vi "ClusterToDescriptiveStringGeneral.vi"(8 "error in":errorcluster, 11 "Cluster In":refnum<vi>) -> (0 "error out":errorcluster, 3 "String":string)   [LabVIEW 2023]
doc: "This VI turns a cluster (from reference) into a human/machine readable string."
panel:
  out "data":dbl[](array[numeric])
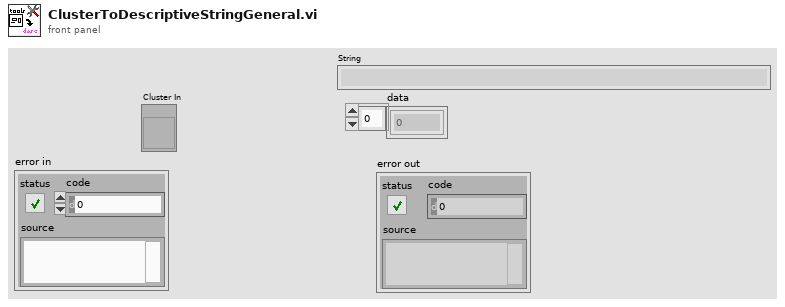
[diagram p1: front panel]
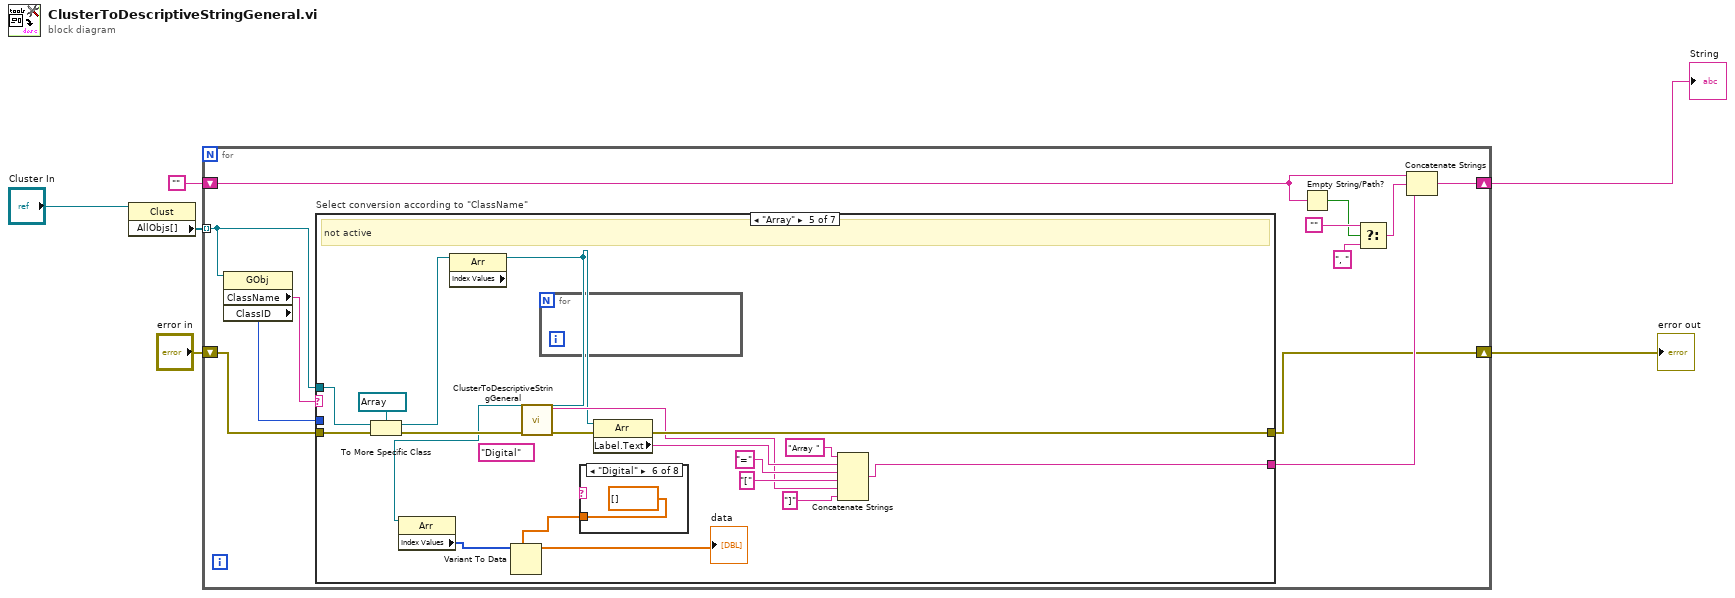
[diagram p0: block diagram]
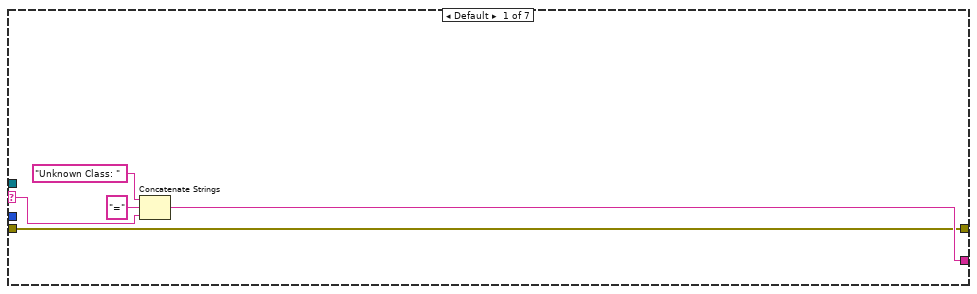
[diagram p2: hidden frame]
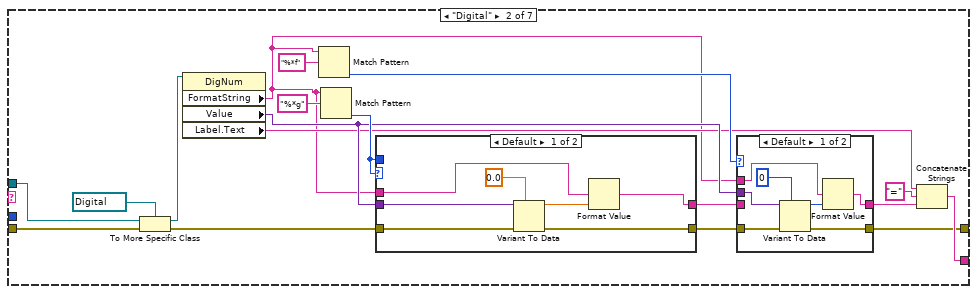
[diagram p3: hidden frame]
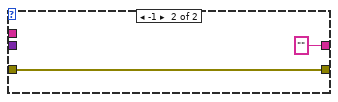
[diagram p5: hidden frame]
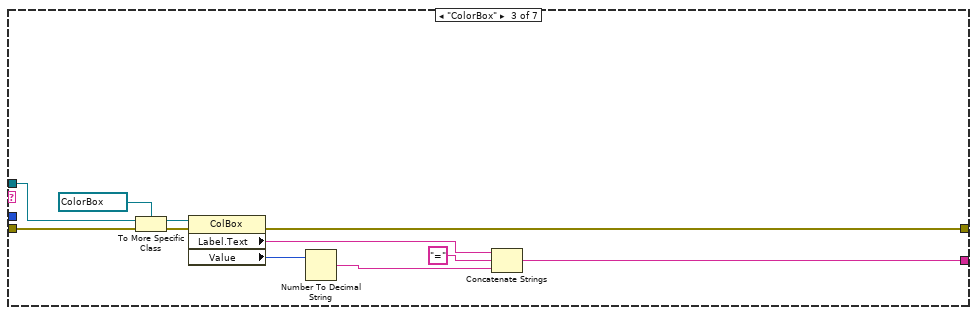
[diagram p6: hidden frame]
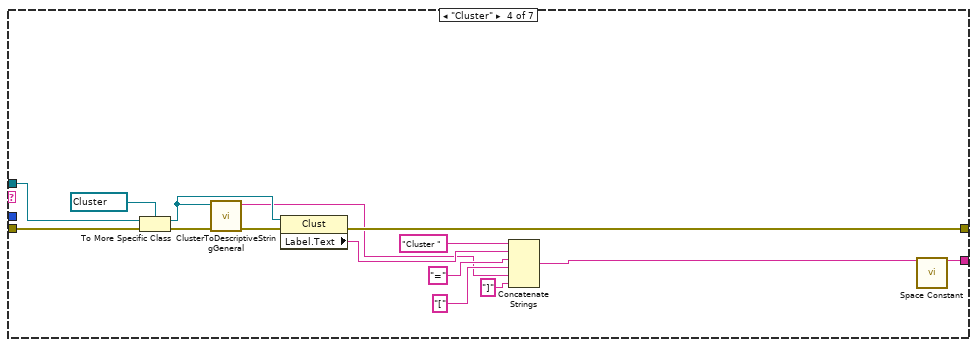
[diagram p7: hidden frame]
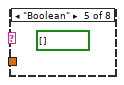
[diagram p12: hidden frame]
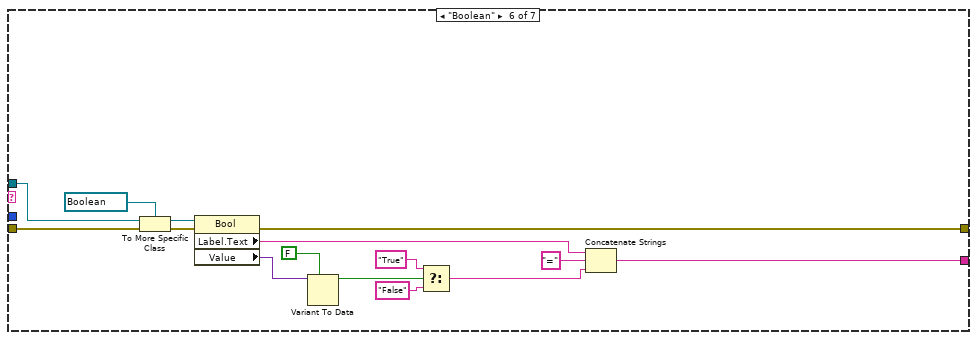
[diagram p15: hidden frame]
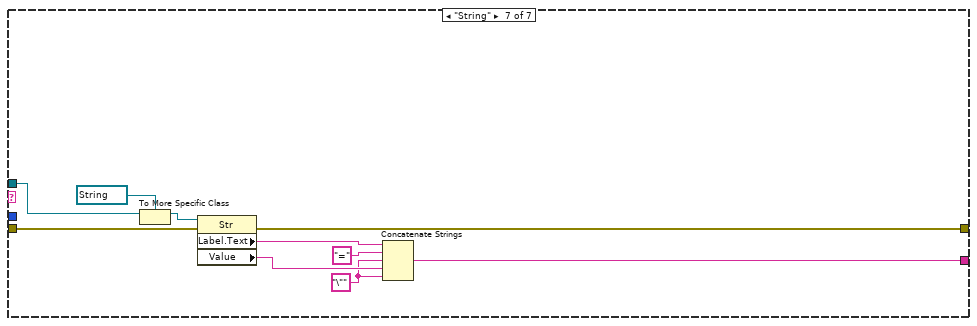
[diagram p16: hidden frame]
diagram:
  n1 = property on="Property Node" class="Clust"(reference="Cluster In") -> ("AllObjs[]"=w2:refnum<vi>[])  [unwired: 1 in, 2 out]
  n2 = for {
    tunnel: w2 -> [w17] mode=indexing
    shift-right: [w18] -> w6
    shift-left: "" ("Empty String Constant") -> [w8]
    shift-right: [w11] -> w3
    shift-left: "error in" -> [w10]
    n3 = property on="Property Node" class="GObj"(reference=w17) -> ("ClassName"=w15:string, "ClassID"=w16:u32)  [unwired: 1 in, 2 out]
    n4 = case "Select conversion according to \"ClassName\"" shown="\"Array\"" w15 {
      selector: w15 -> [w21 _ _ _ _ _ _]
      tunnel: [w20 w31 w66 w82 w100 w115 w126] -> w14
      tunnel: w17 -> [_ w41 w70 w84 w102 w118 w128]
      tunnel: w16 -> [_ _ _ _ _ _ _]
      tunnel: [w19 w25 w62 w79 w98 w106 w120] -> w11
      tunnel: w10 -> [w19 w28 w60 w78 w97 w104 w119]
      frame Default {
        n5 = Concatenate Strings("Unknown Class: ", "=", w21) -> (w20:string)
      }
      frame "Digital" {
        n6 = To More Specific Class(target class=refnum<vi> refnum ("567"), reference=w41, error in=w28) -> (specific class reference=w40:refnum<vi>, error out=w27:errorcluster)
        n7 = property on="Property Node" class="DigNum"(reference=w40) -> ("FormatString"=w30:string, "Value"=w37:variant, "Label.Text"=w33:string)  [unwired: 1 in, 2 out]
        n8 = Match Pattern(string=w30, regular expression="%*f") -> (offset past match=w34:i32)  [unwired: 1 in, 3 out]
        n9 = Match Pattern(string=w30, regular expression="%*g") -> (offset past match=w39:i32)  [unwired: 1 in, 3 out]
        n10 = case shown="Default" w39 {
          tunnel: w39 -> [_ _]
          tunnel: w37 -> [w57 _]
          tunnel: [w55 "" ("output string")] -> w38
          tunnel: w30 -> [w54 _]
          tunnel: w27 -> [w53 w58]
          tunnel: [w52 w58] -> w26
          frame Default {
            n11 = Variant To Data(error in=w53, type=0.0, Variant=w57) -> (data=w56:dbl, error out=w52:errorcluster)
            n12 = Format Value(format string=w54, value (0)=w56) -> (output string=w55:string)  [unwired: 1 in]
          }
          frame -1 {
          }
        }
        n13 = case shown="Default" w34 {
          tunnel: w37 -> [w48 _]
          tunnel: w38 -> [_ w50]
          tunnel: [w46 w50] -> w32
          tunnel: w30 -> [w45 _]
          tunnel: w26 -> [w44 w49]
          tunnel: [w43 w49] -> w25
          frame Default {
            n14 = Variant To Data(error in=w44, type=0, Variant=w48) -> (data=w47:i32, error out=w43:errorcluster)
            n15 = Format Value(format string=w45, value (0)=w47) -> (output string=w46:string)  [unwired: 1 in]
          }
          frame -1 {
          }
        }
        n16 = Concatenate Strings(w33, "=" ("string"), w32) -> (w31:string)
      }
      frame "ColorBox" {
        n17 = To More Specific Class(target class=refnum<vi> refnum ("Left"), reference=w70, error in=w60) -> (specific class reference=w69:refnum<vi>, error out=w61:errorcluster)
        n18 = property on="Property Node" class="ColBox"(reference=w69, error in=w61) -> (error out=w62:errorcluster, "Label.Text"=w67:string, "Value"=w64:u32)  [unwired: 1 out]
        n19 = Number To Decimal String(number=w64) -> (decimal integer string=w68:string)  [unwired: 1 in]
        n20 = Concatenate Strings(w67, "=" ("string"), w68) -> (w66:string)
      }
      frame "Cluster" {
        n21 = To More Specific Class(target class=refnum<vi> refnum ("Left"), reference=w84, error in=w78) -> (specific class reference=w76:refnum<vi>, error out=w77:errorcluster)
        n22 = call "ClusterToDescriptiveStringGeneral.vi"("error in"=w77, "Cluster In"=w76) -> ("error out"=w75:errorcluster, "String"=w73:string)  [unwired: 8 in]
        n23 = property on="Property Node" class="Clust"(reference=w76, error in=w75) -> (error out=w79:errorcluster, "Label.Text"=w83:string)  [unwired: 1 out]
        n24 = Concatenate Strings("Cluster " ("string"), w83, "=" ("string"), "[" ("string"), w73, "]" ("string")) -> (w82:string)
        n25 = call <vilib>:"Space Constant.vi"() -> ()  [unwired: 1 out]
      }
      frame "Array" {
        (unwired) "Digital" ("Combo Box")
        # "not active"
        n26 = To More Specific Class(target class=refnum<vi> refnum ("Left"), reference=w102, error in=w97) -> (specific class reference=w89:refnum<vi>, error out=w96:errorcluster)
        n27 = property on="Property Node" class="Arr" props=["Index Values"](reference=w89) -> (reference out=w88:refnum<vi>)  [unwired: 1 in, 2 out]
        n28 = property on="Property Node" class="Arr"(reference=w88) -> ("Index Values"=w87:u32[])  [unwired: 1 in, 2 out]
        n29 = call "ClusterToDescriptiveStringGeneral.vi"("error in"=w96) -> ("error out"=w95:errorcluster, "String"=w93:string)  [unwired: 9 in]
        n30 = for {
        }
        n31 = case shown="\"Digital\"" {
          selector: _ -> [_ _ _ _ _ _ _ _]
          tunnel: [_ _ _ _ _ dbl[] [] _ _] -> w86
          frame "False", Default {
          }
          frame "True" {
          }
          frame "String" {
          }
          frame "ColorBox" {
          }
          frame "Boolean" {
            (unwired) bool[] []
          }
          frame "Digital" {
          }
          frame "Array" {
          }
          frame "Cluster" {
          }
        }
        n32 = Variant To Data(type=w86, Variant=w87) -> (data=→"data":dbl[])  [unwired: 1 in, 1 out]
        n33 = property on="Property Node" class="Arr"(reference=w88, error in=w95) -> (error out=w98:errorcluster, "Label.Text"=w101:string)  [unwired: 1 out]
        n34 = Concatenate Strings("Array " ("string"), w101, "=" ("string"), "[" ("string"), w93, "]" ("string")) -> (w100:string)
      }
      frame "Boolean" {
        n35 = To More Specific Class(target class=refnum<vi> refnum ("Left"), reference=w118, error in=w104) -> (specific class reference=w117:refnum<vi>, error out=w105:errorcluster)
        n36 = property on="Property Node" class="Bool"(reference=w117, error in=w105) -> (error out=w106:errorcluster, "Label.Text"=w116:string, "Value"=w112:variant)  [unwired: 1 out]
        n37 = Variant To Data(type=FALSE ("x = y?"), Variant=w112) -> (data=w110:bool)  [unwired: 1 in, 1 out]
        n38 = Select(t="True" ("Label.Text"), s=w110, f="False" ("Label.Text")) -> (s? t:f=w107:string)
        n39 = Concatenate Strings(w116, "=" ("string"), w107) -> (w115:string)
      }
      frame "String" {
        w123 = "\"" ("string")
        n40 = To More Specific Class(target class=refnum<vi> refnum ("Numeric"), reference=w128) -> (specific class reference=w127:refnum<vi>)  [unwired: 1 in, 1 out]
        n41 = property on="Property Node" class="Str"(reference=w127, error in=w119) -> (error out=w120:errorcluster, "Label.Text"=w122:string, "Value"=w124:string)  [unwired: 1 out]
        n42 = Concatenate Strings(w122, "=" ("string"), w123, w124, w123) -> (w126:string)
      }
    }
    n43 = Empty String/Path?(string/path=w8) -> (empty?=w7:bool)
    n44 = Select(t="" ("Empty String Constant"), s=w7, f=", " ("string")) -> (s? t:f=w12:string)
    n45 = Concatenate Strings(w8, w12, w14) -> (w18:string)
  }
  "String" <- w6
  "error out" <- w3
